vi "Write Graph Dictionary.vi"(8 "error in (no error)":errorcluster, 10 "Graph Dictionary":variant, 11 "Graph in":refnum<class "Graph.lvclass">) -> (0 "error out":errorcluster, 3 "Graph out":refnum<class "Graph.lvclass">)   [LabVIEW 2013, in "Graph.lvclass"]
uses:
  Graph.lvclass
  Graph.lvclass/Graph.ctl
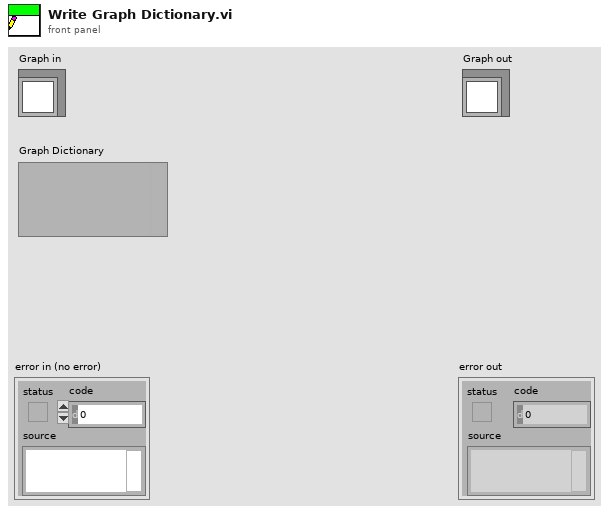
[diagram p1: front panel]
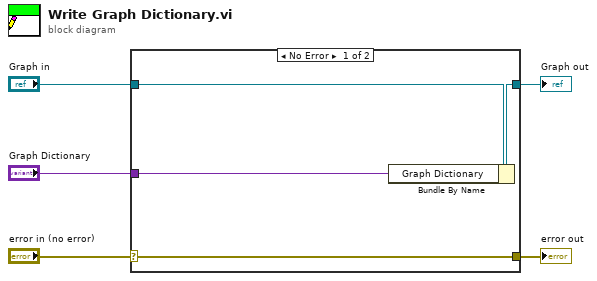
[diagram p0: block diagram]
diagram:
  n1 = case shown="No Error" "error in (no error)" {
    selector: "error in (no error)" -> [w9 w10]
    tunnel: [w9 w10] -> w4
    tunnel: [w7 w11] -> w2
    tunnel: "Graph in" -> [w8 w11]
    tunnel: "Graph Dictionary" -> [w6 _]
    frame No Error {
      n2 = Bundle By Name(cluster=w8, "Graph Dictionary"=w6) -> (w7:refnum<class "Graph.lvclass">)
    }
    frame Error {
    }
  }
  "error out" <- w4
  "Graph out" <- w2
